vi "User32.SendMessageA_num.vi"(0 "HWnd":i32, 5 "Msg":i32, 7 "WParam":i32, 9 "LParam":i32, 11 "ErrorIn":errorcluster) -> (4 "HWndOut":i32, 15 "ErrorOut":errorcluster)   [LabVIEW 2021]
uses:
  user32.dll
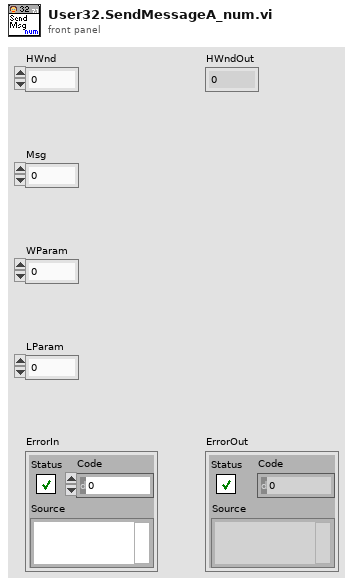
[diagram p1: front panel]
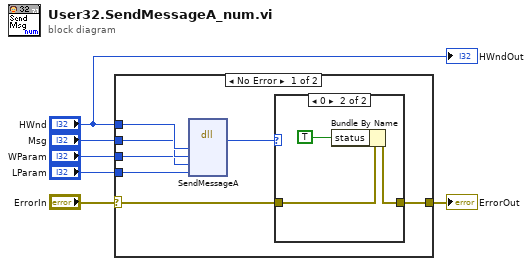
[diagram p0: block diagram]
diagram:
  n1 = case shown="No Error" "ErrorIn" {
    selector: "ErrorIn" -> [w13 w18]
    tunnel: "HWnd" -> [w11 _]
    tunnel: "Msg" -> [w10 _]
    tunnel: "WParam" -> [w9 _]
    tunnel: "LParam" -> [w8 _]
    tunnel: [w12 w18] -> w5
    frame No Error {
      n2 = dll-call lib="user32.dll" fn="SendMessageA"("hWnd"=w11, "Msg"=w10, "wParam"=w9, "lParam"=w8) -> (w7:i32)  [unwired: 7 in, 2 out]
      n3 = case shown="0" w7 {
        tunnel: w13 -> [w14 w17]
        tunnel: [w14 w16] -> w12
        frame Default {
        }
        frame 0 {
          n4 = Bundle By Name(cluster=w17, "status"=TRUE) -> (w16:errorcluster)
        }
      }
    }
    frame Error {
    }
  }
  "ErrorOut" <- w5
  "HWndOut" <- "HWnd"
